vi "Destroy.vi"(8 "error in (no error)":errorcluster, 11 "Mock Report In":refnum<class "Mock Report.lvclass">) -> (0 "error out":errorcluster)   [LabVIEW 2020, in "Mock Report.lvclass"]
uses:
  Mock Report.lvclass
  Mock Report.lvclass/Mock Report.ctl
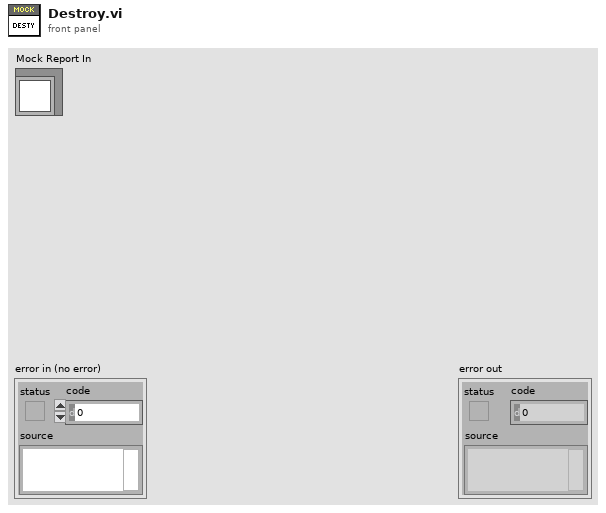
[diagram p1: front panel]
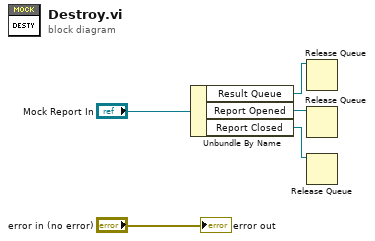
[diagram p0: block diagram]
diagram:
  n1 = Unbundle By Name("Mock Report In") -> ("Result Queue"=w3:refnum<queue>, "Report Opened"=w2:refnum<queue>, "Report Closed"=w1:refnum<queue>)
  n2 = Release Queue(queue=w3) -> ()  [unwired: 2 in, 3 out]
  n3 = Release Queue(queue=w2) -> ()  [unwired: 2 in, 3 out]
  n4 = Release Queue(queue=w1) -> ()  [unwired: 2 in, 3 out]
  "error out" <- "error in (no error)"
